vi "Init.vi"(8 "error in":errorcluster, 10 "Key Name":string, 11 "Key Name in":refnum<class "Key Name.lvclass">) -> (0 "error out":errorcluster, 3 "Key Name out":refnum<class "Key Name.lvclass">)   [LabVIEW 2024, in "EDS.lvlib" / "Key Name.lvclass"]
uses:
  Key Name.lvclass
  Key Name.lvclass/Key Name.ctl
  <vilib>/Utility/error.llb/Trim Whitespace One-Sided.vi
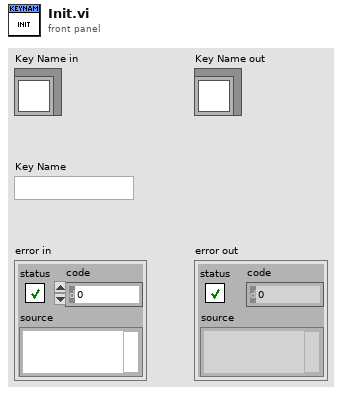
[diagram p1: front panel]
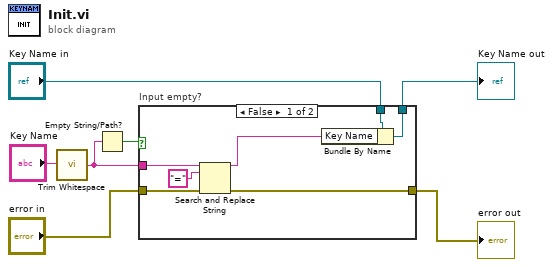
[diagram p0: block diagram]
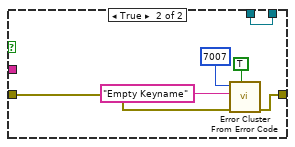
[diagram p2: hidden frame]
diagram:
  n1 = call <vilib>:"Trim Whitespace.vi"("string"="Key Name") -> ("trimmed string"=w2:string)  [unwired: 1 in]
  n2 = Empty String/Path?(string/path=w2) -> (empty?=w1:bool)
  n3 = case "Input empty?" shown="False" w1 {
    tunnel: "error in" -> [w13 w18]
    tunnel: [w12 w20] -> w5
    tunnel: "Key Name in" -> [w11 w19]
    tunnel: [w10 w19] -> w3
    tunnel: w2 -> [w8 _]
    frame False {
      n4 = Search and Replace String(input string=w8, search string="=", error in=w13) -> (result string=w9:string, error out=w12:errorcluster)  [unwired: 5 in, 2 out]
      n5 = Bundle By Name(cluster=w11, "Key Name"=w9) -> (w10:refnum<class "Key Name.lvclass">)
    }
    frame True {
      n6 = call <vilib>:"Error Cluster From Error Code.vi"("show call chain? (False)"=TRUE, "error in (no error)"=w18, "error message (\"\")"="Empty Keyname" ("error message (\"\")"), "error code (0)"=7007) -> ("error out"=w20:errorcluster)  [unwired: 5 in]
    }
  }
  "error out" <- w5
  "Key Name out" <- w3
